vi "Global TeamLeader.vi"() -> ()   [LabVIEW 2020]
panel:
  out "TL?":bool
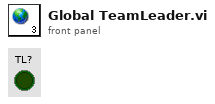
[diagram p1: front panel]
diagram:
